vi "401_Unauthorized.vi"(8 "error in (no error)":errorcluster, 11 "headers":string="HTTP/1.1 401 Unauthorized\r\nWWW-Authenticate: Digest realm=\"Login to 4H0572FPAG801C6\", qop=\"auth\", nonce=\"1763322981\", opaque=\"a663b9f7478c0416c2eaa1c598bca2154a0b27af\"\r\nConnection: close\r\nCONTENT-LENGTH: 0\r\n\r\nHTTP/1.1 400 Bad Request\r\nConnection: close\r\nContent-type: text/plain;charset=utf-8\r\nContent-Length: 21\r\n\r\n") -> (0 "error out":errorcluster, 2 "ServerInfo":T1={"realm"="Login to 4H0572FPAG801C6", "qop"="auth", "nounce"="\u0017c2)", "opaque"="a663b9f7478c0416c2eaa1c598bca2154a0b27af"}, 3 "401?":bool=TRUE)   [LabVIEW 2016]
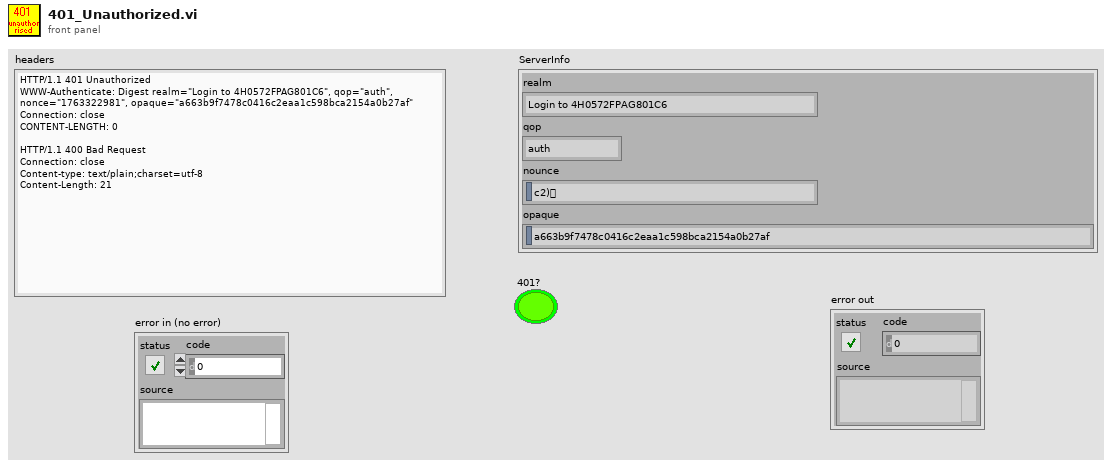
[diagram p1: front panel]
types:
  T1 = cluster{"realm":string, "qop":string, "nounce":string, "opaque":string}
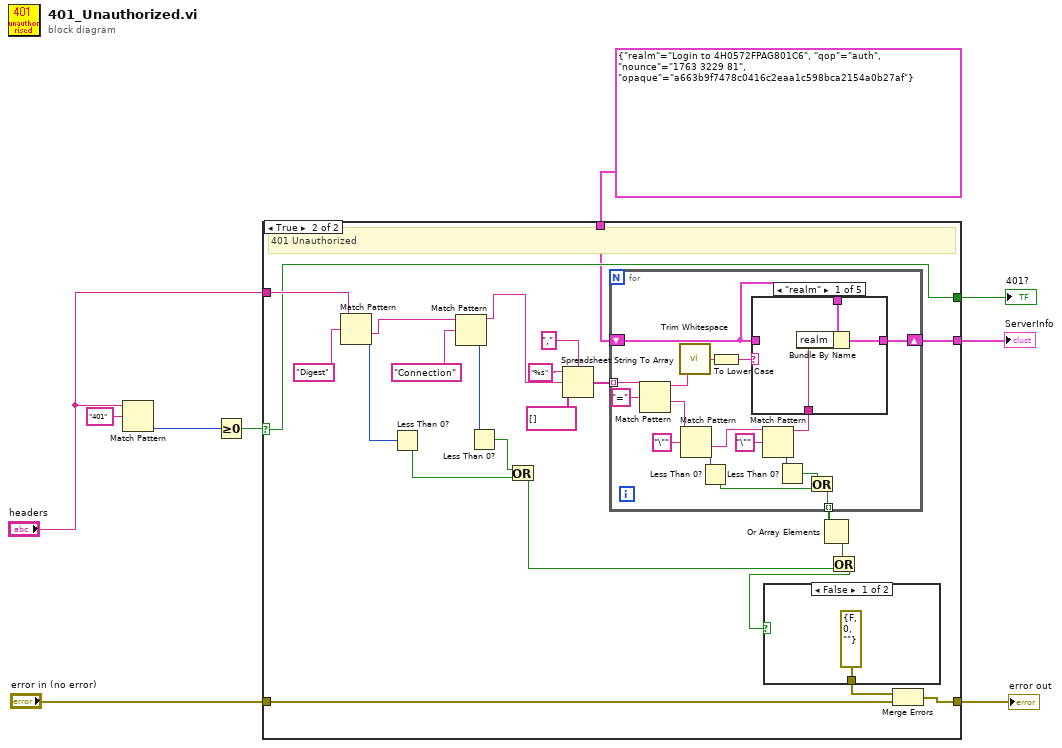
[diagram p0: block diagram]
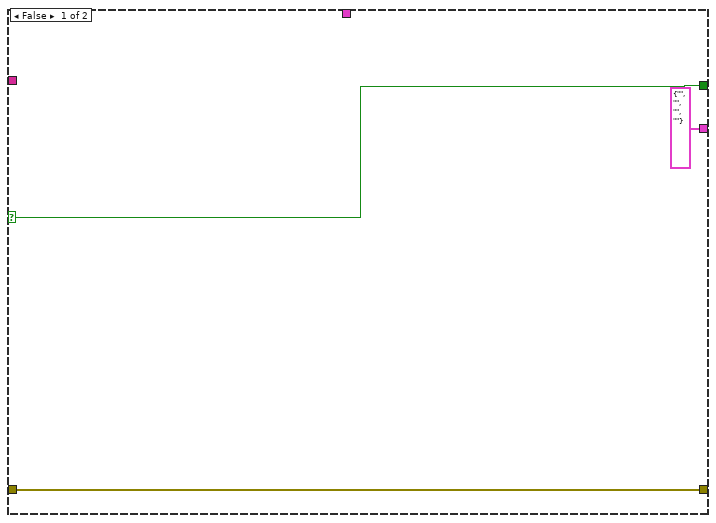
[diagram p2: hidden frame]
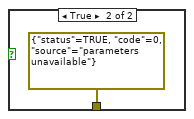
[diagram p3: hidden frame]
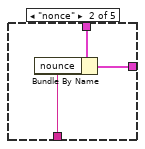
[diagram p4: hidden frame]
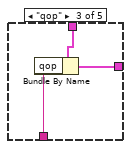
[diagram p5: hidden frame]
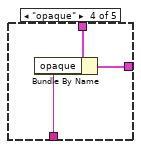
[diagram p6: hidden frame]
diagram:
  n1 = Match Pattern(string="headers", regular expression="401") -> (offset past match=w6:i32)  [unwired: 1 in, 3 out]
  n2 = Greater Or Equal To 0?(x=w6) -> (x >= 0?=w7:bool)
  n3 = case shown="True" w7 {
    selector: w7 -> [w12 w27]
    tunnel: "headers" -> [_ w35]
    tunnel: [w12 w27] -> w5
    tunnel: "error in (no error)" -> [w11 w17]
    tunnel: [w11 w16] -> w3
    tunnel: [T1 {"realm"="", "qop"="", "nounce"="", "opaque"=""} ("ServerInfo") w14] -> w2
    tunnel: T1 {"realm"="Login to 4H0572FPAG801C6", "qop"="auth", "nounce"="1763 3229 81", "opaque"="a663b9f7478c0416c2eaa1c598bca2154a0b27af"} ("ServerInfo") -> [_ w13]
    frame False {
    }
    frame True {
      # "401 Unauthorized"
      n4 = Match Pattern(string=w35, regular expression="Digest") -> (after substring=w26:string, offset past match=w25:i32)  [unwired: 1 in, 2 out]
      n5 = Less Than 0?(x=w25) -> (x < 0?=w21:bool)
      n6 = Match Pattern(string=w26, regular expression="Connection") -> (before substring=w29:string, offset past match=w24:i32)  [unwired: 1 in, 2 out]
      n7 = Less Than 0?(x=w24) -> (x < 0?=w22:bool)
      n8 = Or(x=w22, y=w21) -> (x .or. y?=w19:bool)
      n9 = Spreadsheet String To Array(delimiter (Tab)=",", format string="%s", spreadsheet string=w29, array type (2D Dbl)=string[] [] ("Array Constant")) -> (array=w28:string[])
      n10 = for {
        tunnel: w28 -> [w53] mode=indexing
        tunnel: [w44] -> w23 mode=indexing
        shift-right: [w39] -> w14
        shift-left: w13 -> [w38]
        n11 = Match Pattern(string=w53, regular expression="=") -> (before substring=w43:string, after substring=w52:string)  [unwired: 1 in, 2 out]
        n12 = call <vilib>:"Trim Whitespace.vi"("string"=w43) -> ("trimmed string"=w42:string)  [unwired: 1 in]
        n13 = Match Pattern(string=w52, regular expression="\"") -> (after substring=w50:string, offset past match=w48:i32)  [unwired: 1 in, 2 out]
        n14 = Less Than 0?(x=w48) -> (x < 0?=w45:bool)
        n15 = To Lower Case(string=w42) -> (all lower case string=w41:string)
        n16 = Match Pattern(string=w50, regular expression="\"") -> (before substring=w40:string, offset past match=w47:i32)  [unwired: 1 in, 2 out]
        n17 = case shown="\"realm\"" w41 {
          tunnel: w38 -> [w57 w60 w63 w66 _]
          tunnel: w40 -> [w55 w59 w62 w65 _]
          tunnel: [w56 w58 w61 w64 w67] -> w39
          tunnel: w38 -> [_ _ _ _ w67]
          frame "realm" {
            n18 = Bundle By Name(cluster=w57, "realm"=w55) -> (w56:T1)
          }
          frame "nonce" {
            n19 = Bundle By Name(cluster=w60, "nounce"=w59) -> (w58:T1)
          }
          frame "qop" {
            n20 = Bundle By Name(cluster=w63, "qop"=w62) -> (w61:T1)
          }
          frame "opaque" {
            n21 = Bundle By Name(cluster=w66, "opaque"=w65) -> (w64:T1)
          }
          frame Default {
          }
        }
        n22 = Less Than 0?(x=w47) -> (x < 0?=w46:bool)
        n23 = Or(x=w46, y=w45) -> (x .or. y?=w44:bool)
      }
      n24 = Or Array Elements(Boolean array=w23) -> (logical OR=w20:bool)
      n25 = Or(x=w20, y=w19) -> (x .or. y?=w18:bool)
      n26 = case shown="False" w18 {
        tunnel: [errorcluster {"status"=FALSE, "code"=0, "source"=""} ("error constant") errorcluster {"status"=TRUE, "code"=0, "source"="parameters unavailable"} ("error constant")] -> w15
        frame False {
        }
        frame True {
        }
      }
      n27 = Merge Errors(w15, w17) -> (w16:errorcluster)
    }
  }
  "401?" <- w5
  "error out" <- w3
  "ServerInfo" <- w2
